vi "CLAD try.vi"() -> ()   [LabVIEW 2020]
panel:
  out "array w/ subset deleted 2":i32[](array[numeric])
  out "deleted portion 2":i32[](array[numeric])
  out "deleted portion":i32[](array[numeric])
  out "array w/ subset deleted":i32[](array[numeric])
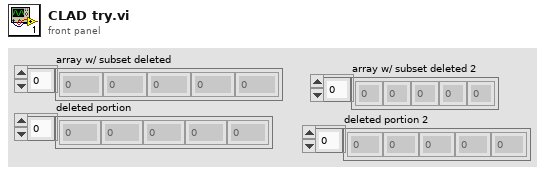
[diagram p1: front panel]
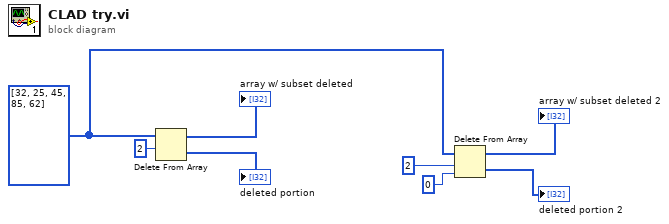
[diagram p0: block diagram]
diagram:
  w1 = i32[] [32, 25, 45, 85, 62]
  n1 = Delete From Array "Delete From Array"(array=w1, length=2) -> (deleted portion=→"deleted portion":i32[], array with subset deleted=→"array w/ subset deleted":i32[])  [unwired: 1 in]
  n2 = Delete From Array "Delete From Array"(array=w1, length=2, index=0 ("length")) -> (deleted portion=→"deleted portion 2":i32[], array with subset deleted=→"array w/ subset deleted 2":i32[])
